vi "Read all parameters.vi"() -> ()   [LabVIEW 2021, in "F-70 driver.lvlib"]
uses:
  F-70 driver.lvlib
  Commands.ctl
  F-70 parameters.ctl
panel:
  out "Checksum OK":bool
  out "VISA resource name out":refnum<visa-resource-name>
  out "F-70 parameters in 2":T1 {"Last updated" format="%<%d/%m/%Y %H:%M:%S>T"; "State of operation" items=["Local Off", "Local On", "Remote Off", "Remote On", "Cold head Run", "Cold head pause", "Fault Off", "Oil Fault Off"]; "Return pressure (PSIG)" scale=0.0..200.0; "Water in Tmp (°C)" scale=0.0..100.0; "Water out Tmp (°C)" scale=0.0..100.0; "He discharge Tmp (°C)" scale=0.0..100.0}
  in  "VISA resource name":refnum<visa-resource-name>
  in  "F-70 parameters in":T1 {"Last updated" format="%<%d/%m/%Y %H:%M:%S>T"; "State of operation" items=["Local Off", "Local On", "Remote Off", "Remote On", "Cold head Run", "Cold head pause", "Fault Off", "Oil Fault Off"]; "Return pressure (PSIG)" scale=0.0..200.0; "Water in Tmp (°C)" scale=0.0..100.0; "Water out Tmp (°C)" scale=0.0..100.0; "He discharge Tmp (°C)" scale=0.0..100.0}
  out "error out":errorcluster
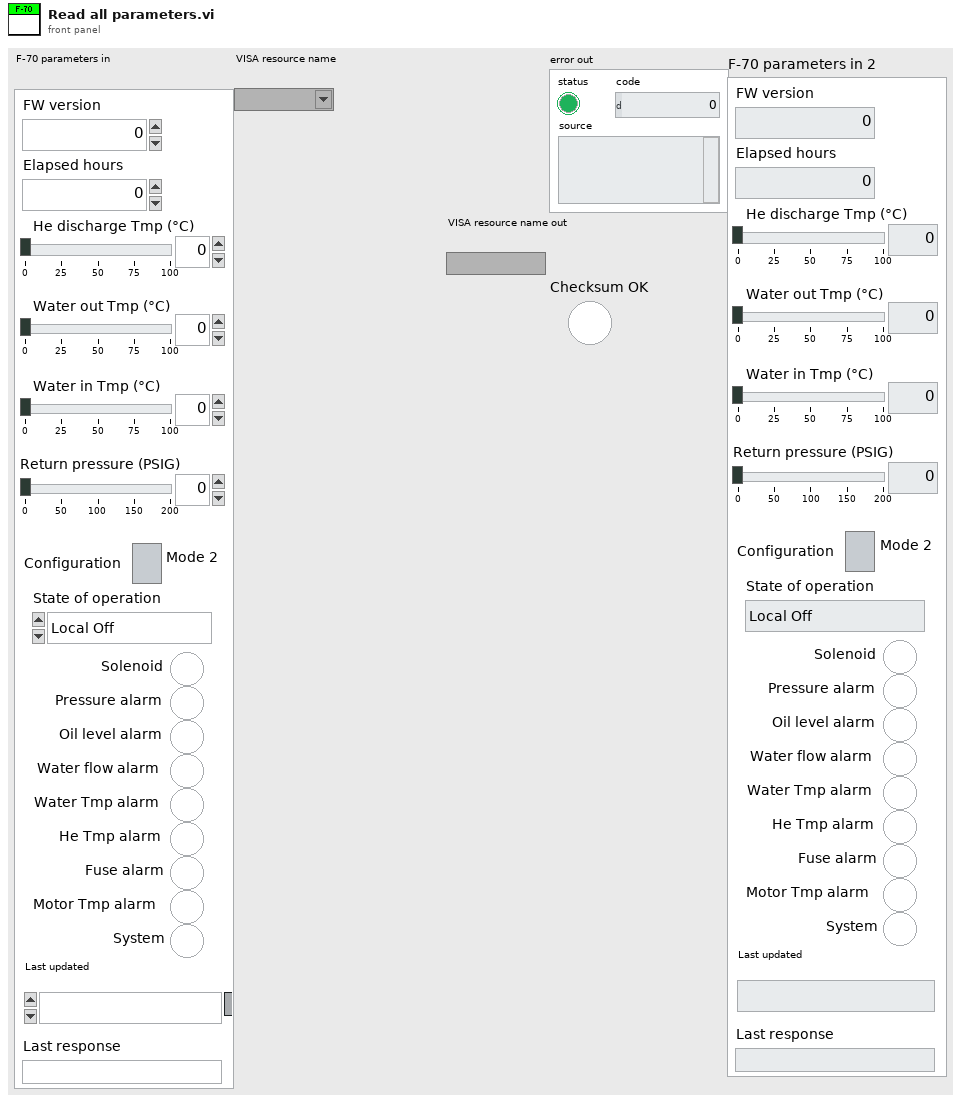
[diagram p1: front panel]
types:
  T1 = typedef "F-70 driver.lvlib/F-70 parameters.ctl" = cluster{"FW version":dbl, "Elapsed hours":dbl, "He discharge Tmp (°C)":dbl, "Water out Tmp (°C)":dbl, "Water in Tmp (°C)":dbl, "Return pressure (PSIG)":dbl, "Configuration":bool, "State of operation":u16, "Solenoid":bool, "Pressure alarm":bool, "Oil level alarm":bool, "Water flow alarm":bool, "Water Tmp alarm":bool, "He Tmp alarm":bool, "Fuse alarm":bool, "Motor Tmp alarm":bool, "System":bool, "Last updated":timestamp, "Last response":string}
  T2 = typedef "F-70 driver.lvlib/Commands.ctl" = enum16{"TEA", "PRA", "STA", "ID1", "ON1", "RS1", "CHP", "OFF", "CHR", "POF"}
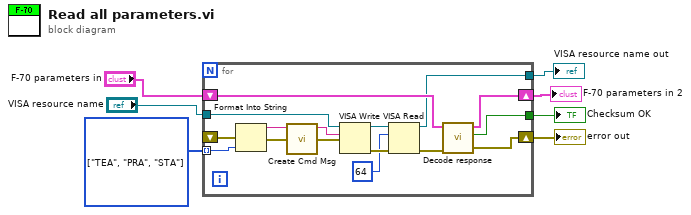
[diagram p0: block diagram]
diagram:
  w7 = T2[] [enum."TEA", enum."PRA", enum."STA"] items=["TEA", "PRA", "STA", "ID1", "ON1", "RS1", "CHP", "OFF", "CHR", "POF"] ("Array")
  n1 = for {
    tunnel: w7 -> [w22] mode=indexing
    shift-right: [w15] -> w3
    shift-left: "F-70 parameters in" -> [w16]
    tunnel: "VISA resource name" -> [w13]
    shift-right: [w17] -> w6
    shift-left: _ -> [w12]
    tunnel: [w9] -> w2
    tunnel: [w8] -> w1
    n2 = Format Into String(error in=w12, w22) -> (resulting string=w21:string, error out=w20:errorcluster)  [unwired: 2 in]
    n3 = call "Create Cmd Msg.vi"("command"=w21) -> ("complete message"=w14:string)  [unwired: 10 in]
    n4 = VISA Write(VISA resource name=w13, write buffer=w14, error in (no error)=w20) -> (VISA resource name out=w11:refnum<visa-resource-name>, error out=w19:errorcluster)  [unwired: 1 out]
    n5 = VISA Read(VISA resource name=w11, byte count=u32 64, error in (no error)=w19) -> (VISA resource name out=w9:refnum<visa-resource-name>, error out=w18:errorcluster)  [unwired: 2 out]
    n6 = call "Decode response.vi"("error in"=w18, "F-70 parameters in"=w16) -> ("error out"=w17:errorcluster, "Checksum OK"=w8:bool, "F-70 parameters out"=w15:T1)  [unwired: 7 in]
  }
  "error out" <- w6
  "F-70 parameters in 2" <- w3
  "VISA resource name out" <- w2
  "Checksum OK" <- w1
